vi "Main.vi"() -> ()   [LabVIEW 2019]
uses:
  Typedefs/#enum_State.ctl
  <vilib>/sound2/lvsound2.llb/Sound Data Format.ctl
  <vilib>/sound2/lvsound2.llb/Sampling Mode.ctl
  Typedefs/#cluster_ApplicationData.ctl
  <vilib>/sound2/lvsound2.llb/Sound File Refnum.ctl
  <vilib>/sound2/lvsound2.llb/Sound Input Task ID.ctl
  <vilib>/Utility/sysdir.llb/System Directory Type.ctl
  <vilib>/sound2/lvsound2.llb/Sound Input Read (DBL).vi
panel:
  in  "Record":bool
  out "Raw Data":waveform(dbl)[](graph)
  out "Spectrum Data":cluster{"f0":dbl, "df":dbl, "magnitude":dbl[]}[](graph)
  out "Threshold Exceeded?":bool
  in  "Threshold, dB":dbl=-100.0 format="%#_13g"
  in  "Upper Fc":dbl=3500.0 format="%#_13g"
  in  "Lower Fc":dbl=300.0 format="%#_13g"
  in  "Order":i32=6
  in  "Type":T1(ring)
  in  "Stop":bool
  # "FILTER SETTINGS"
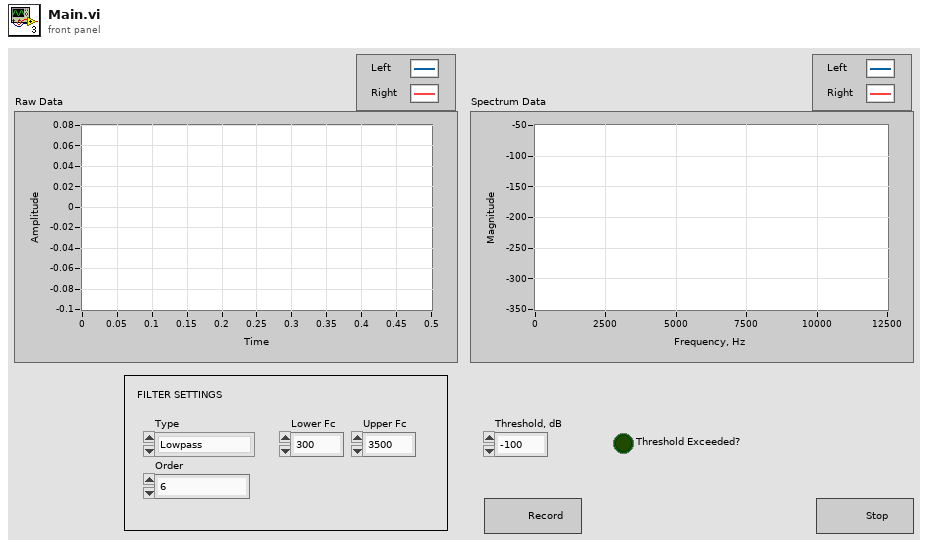
[diagram p1: front panel]
types:
  T1 = enum16{"Lowpass", "Highpass", "Bandpass", "Bandstop"}
  T2 = typedef "#enum_State.ctl" = enum16{"Init", "Acquisition", "Error Handler", "Exit", "Idle"}
  T3 = enum16{"open", "replace", "create", "open or create", "replace or create", "replace or create with confirmation"}
  T4 = typedef "Sound Data Format.ctl" = cluster{"sample rate (S/s)":dbl, "number of channels":i32, "bits per sample":i32}
  T5 = typedef "#cluster_ApplicationData.ctl" = cluster{"Sound file refnum":T6, "Acquisition task ID":T7, "Sound format":T4, "Number of samples/channel":i32, "Logging file refnum":refnum<file>}
  T6 = typedef "Sound File Refnum.ctl" = refnum<file>
  T7 = typedef "Sound Input Task ID.ctl" = u32
  T8 = typedef "System Directory Type.ctl" = i32
  T9 = typedef "Sampling Mode.ctl" = i32
  T10 = cluster{"Topology":enum16{"Off", "Butterworth", "Chebyshev", "Inverse Chebyshev", "Elliptic", "Bessel"}, "Type":enum16{"Lowpass", "Highpass", "Bandpass", "Bandstop"}, "Order":i32, "Lower Fc":dbl, "Upper Fc":dbl, "PB Ripple":dbl, "SB Attenuation":dbl}
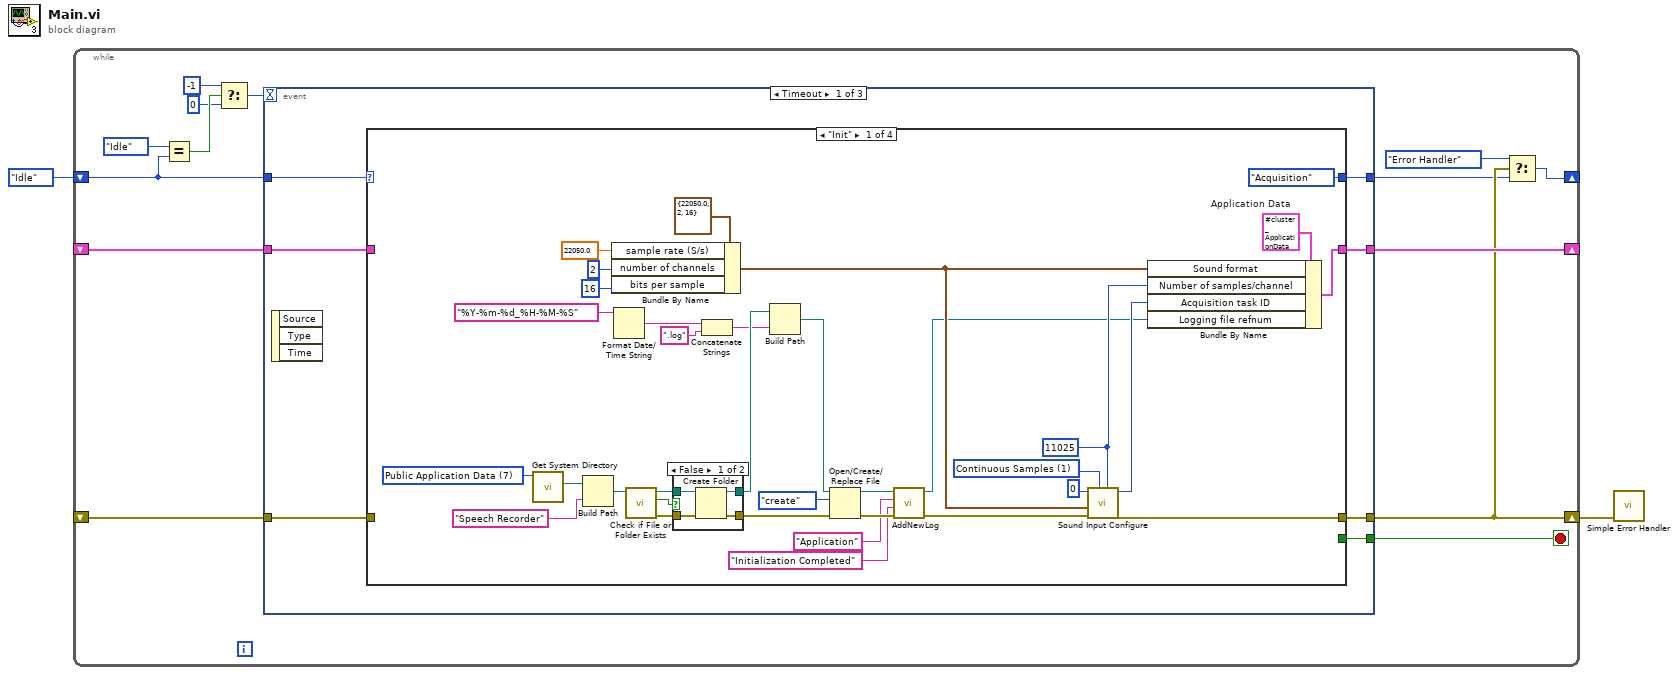
[diagram p0: block diagram]
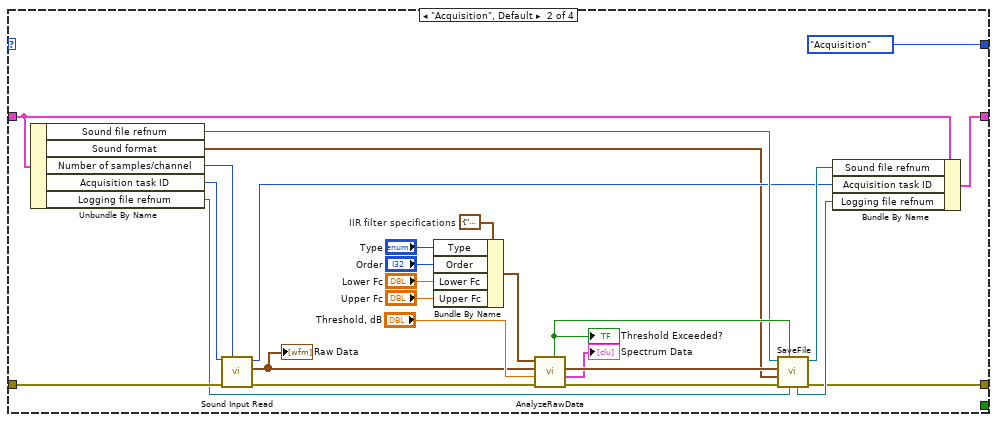
[diagram p3: hidden frame]
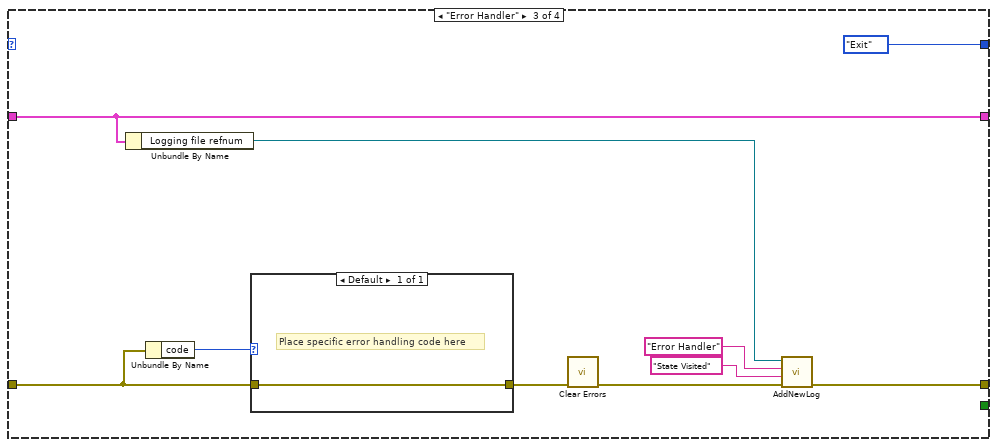
[diagram p4: hidden frame]
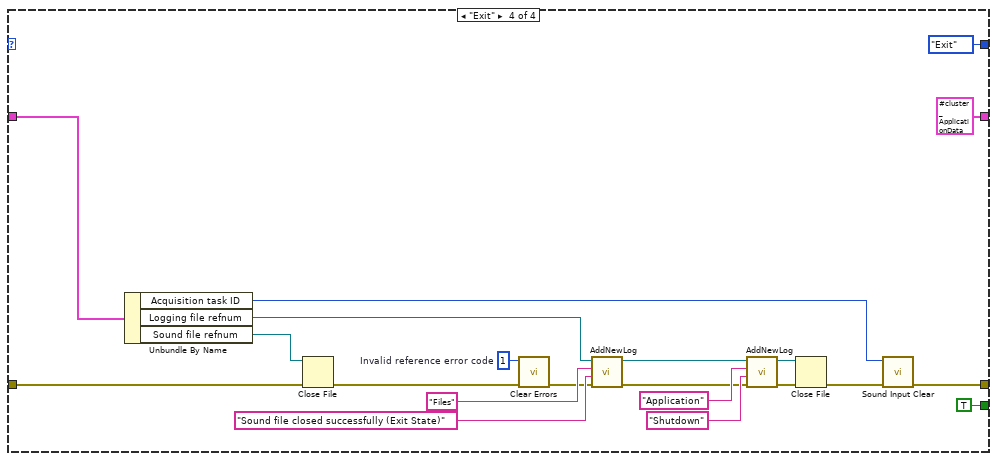
[diagram p5: hidden frame]
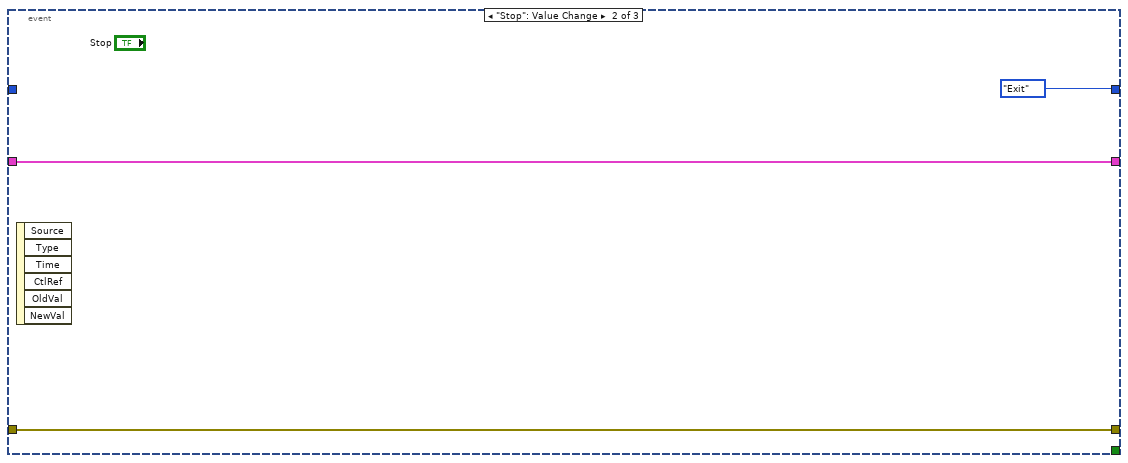
[diagram p6: hidden frame]
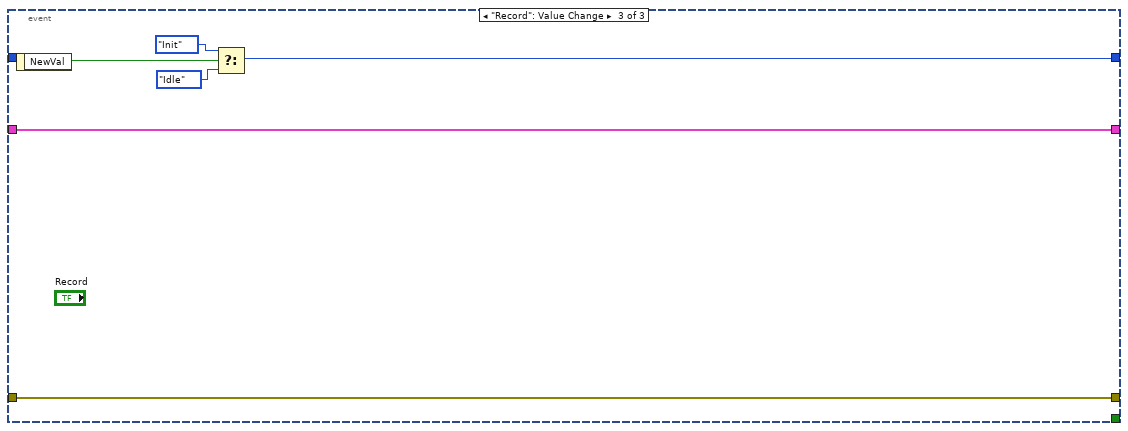
[diagram p7: hidden frame]
diagram:
  n1 = while {
    shift-right: [w9] -> _
    shift-left: #enum_State."Idle" ("State") -> [w8]
    shift-right: [w15] -> _
    shift-left: _ -> [w16]
    shift-right: [w12] -> w2
    shift-left: _ -> [w14]
    stop <- w13 stop-if-true
    n2 = Equal?(x=#enum_State."Idle", y=w8) -> (x = y?=w6:bool)
    n3 = Select(t=-1, s=w6, f=0) -> (s? t:f=w3:i32)
    n4 = event shown="[0] Timeout" {
      selector: _ -> [_ _ _]
      dyn-events: _ -> [_ _ _]
      timeout: w3 -> [_ _ _]
      tunnel: w8 -> [w23 _ _]
      tunnel: w16 -> [w22 w124 w130]
      tunnel: [w21 w124 w130] -> w15
      tunnel: w14 -> [w20 w123 w129]
      tunnel: [w19 _ _] -> w13
      tunnel: [w18 w123 w129] -> w12
      tunnel: [w17 #enum_State."Exit" ("State") w125] -> w10
      event Timeout {
        n5 = event-data() -> ()  [unwired: 1 in, 3 out]
        n6 = case shown="\"Init\"" w23 {
          tunnel: w20 -> [_ w89 w90 w121]
          tunnel: [w24 w64 w97 w104] -> w18
          tunnel: w22 -> [_ w74 w94 w118]
          tunnel: [w50 w73 w94 T5 {"Sound file refnum"=refnum, "Acquisition task ID"=0, "Sound format"={"sample rate (S/s)"=22050.0, "number of channels"=2, "bits per sample"=16}, "Number of samples/channel"=0, "Logging file refnum"=refnum} ("Application Data")] -> w21
          tunnel: [#enum_State."Acquisition" ("State") #enum_State."Acquisition" ("State") #enum_State."Exit" ("State") #enum_State."Exit" ("State")] -> w17
          tunnel: [_ _ _ TRUE] -> w19
          frame "Init" {
            w45 = T8 7 items=["User Home"=0, "User Desktop"=1, "User Documents"=2, "User Application Data"=3, "User Preferences"=4, "User Temporary"=5, "Public Documents"=6, "Public Application Data"=7, "Public Preferences"=8, "Public Cache"=13, "System Core Libraries"=9, "System Installed Libraries"=10, "Application Files"=11, "Boot Volume Root"=12] ("system directory type")
            w51 = T5 {"Sound file refnum"=refnum, "Acquisition task ID"=0, "Sound format"={"sample rate (S/s)"=22050.0, "number of channels"=2, "bits per sample"=16}, "Number of samples/channel"=0, "Logging file refnum"=refnum}  # Application Data
            w47 = 11025 ("Number of Samples/ch")
            w57 = T9 1 items=["Finite Samples", "Continuous Samples"] ("sample mode")
            n7 = call <vilib>:"Get System Directory.vi"("system directory type"=w45) -> ("system directory"=w44:path)  [unwired: 10 in]
            n8 = Build Path(base path=w44, name or relative path="Speech Recorder") -> (appended path=w42:path)
            n9 = Bundle By Name(cluster=T4 {"sample rate (S/s)"=22050.0, "number of channels"=2, "bits per sample"=16} ("sound format"), "sample rate (S/s)"=22050.0 ("Sample rate (Hz)"), "number of channels"=2 ("#Channels"), "bits per sample"=16 ("Resolution (bits)")) -> (w49:T4)
            n10 = Format Date/Time String(time format string (%c)="%Y-%m-%d_%H-%M-%S") -> (date/time string=w37:string)  [unwired: 2 in]
            n11 = call <vilib>:"Check if File or Folder Exists.vi"("path"=w42) -> ("error out"=w41:errorcluster, "file or folder exists?"=w39:bool, "dup path"=w40:path)  [unwired: 8 in]
            n12 = case shown="False" w39 {
              tunnel: w41 -> [w61 w62]
              tunnel: [w60 w62] -> w32
              tunnel: w40 -> [w59 w63]
              tunnel: [w58 w63] -> w38
              frame False {
                n13 = Create Folder(path (use dialog)=w59, error in=w61) -> (created path=w58:path, error out=w60:errorcluster)  [unwired: 1 in, 1 out]
              }
              frame True {
              }
            }
            n14 = Concatenate Strings(w37, ".log" ("string")) -> (w34:string)
            n15 = Build Path(base path=w38, name or relative path=w34) -> (appended path=w31:path)
            n16 = Open/Create/Replace File(file path (use dialog)=w31, error in=w32, operation (0:open)=T3."create") -> (refnum out=w28:refnum<file>, error out=w30:errorcluster)  [unwired: 3 in, 1 out]
            n17 = call "AddNewLog.vi"("error in"=w30, "Details"="Initialization Completed", "General Info"="Application", "Logging file refnum in"=w28) -> ("error out"=w29:errorcluster, "Logging file refnum out"=w27:refnum<file>)  [unwired: 6 in]
            n18 = call <vilib>:"Sound Input Configure.vi"("number of samples/ch"=w47, "sample mode"=w57, "error in (no error)"=w29, "sound format"=w49, "device ID"=u32 0 ("Device")) -> ("error out"=w24:errorcluster, "task ID"=w48:T7)  [unwired: 5 in]
            n19 = Bundle By Name(cluster=w51, "Sound format"=w49, "Number of samples/channel"=w47, "Acquisition task ID"=w48, "Logging file refnum"=w27) -> (w50:T5)
          }
          frame "Acquisition", Default {
            w88 = T10 {"Topology"=enum."Butterworth", "Type"=enum."Lowpass", "Order"=1, "Lower Fc"=100.0, "Upper Fc"=200.0, "PB Ripple"=1.0, "SB Attenuation"=60.0}  # IIR filter specifications
            n20 = Unbundle By Name(w74) -> ("Sound file refnum"=w75:T6, "Sound format"=w68:T4, "Number of samples/channel"=w69:i32, "Acquisition task ID"=w70:T7, "Logging file refnum"=w65:refnum<file>)
            n21 = call-poly <vilib>:"Sound Input Read.vi"("number of samples/ch"=w69, "error in (no error)"=w89, "task ID"=w70) -> ("error out"=w83:errorcluster, "data"=w81:waveform(dbl)[], "task ID out"=w71:T7)  [unwired: 6 in]
            "Raw Data" <- w81
            n22 = Bundle By Name(cluster=w88, "Type"="Type", "Order"="Order", "Lower Fc"="Lower Fc", "Upper Fc"="Upper Fc") -> (w80:T10)
            n23 = call "AnalyzeRawData.vi"("error in (no error)"=w83, "Threshold, dB"="Threshold, dB", "Raw Data"=w81, "IIR Filter Specifications"=w80) -> ("error out"=w77:errorcluster, "Power Spectrum / PSD"=→"Spectrum Data":cluster{"f0":dbl, "df":dbl, "magnitude":dbl[]}[], "Filtered Data"=w79:waveform(dbl)[], "Threshold Exceeded?"=w76:bool)  [unwired: 4 in]
            "Threshold Exceeded?" <- w76
            n24 = call "SaveFile.vi"("Logging file refnum in"=w65, "Threshold Exceeded?"=w76, "Error in"=w77, "Sound format"=w68, "Filtered Data"=w79, "Sound file refnum in"=w75) -> ("Error out"=w64:errorcluster, "Sound file refnum out"=w72:T6, "Logging file refnum out"=w66:refnum<file>)  [unwired: 3 in]
            n25 = Bundle By Name(cluster=w74, "Sound file refnum"=w72, "Acquisition task ID"=w71, "Logging file refnum"=w66) -> (w73:T5)
          }
          frame "Error Handler" {
            n26 = Unbundle By Name(w94) -> ("Logging file refnum"=w93:refnum<file>)
            n27 = Unbundle By Name(w90) -> ("code"=w92:i32)
            n28 = case shown="Default" w92 {
              tunnel: [w100] -> w91
              tunnel: w90 -> [w100]
              frame Default {
                # "Place specific error handling code here"
              }
            }
            n29 = call <vilib>:"Clear Errors.vi"("error in (no error)"=w91) -> ("error out"=w99:errorcluster)  [unwired: 5 in, 1 out]
            n30 = call "AddNewLog.vi"("error in"=w99, "Details"="State Visited" ("string"), "General Info"="Error Handler" ("string"), "Logging file refnum in"=w93) -> ("error out"=w97:errorcluster)  [unwired: 6 in, 1 out]
          }
          frame "Exit" {
            w101 = 1  # Invalid reference error code
            n31 = Unbundle By Name(w118) -> ("Acquisition task ID"=w106:T7, "Logging file refnum"=w110:refnum<file>, "Sound file refnum"=w111:T6)
            n32 = Close File(refnum=w111, error in=w121) -> (error out=w103:errorcluster)  [unwired: 1 out]
            n33 = call <vilib>:"Clear Errors.vi"("error in (no error)"=w103, "specific error code to clear (0: all)"=w101) -> ("error out"=w102:errorcluster)  [unwired: 4 in, 1 out]
            n34 = call "AddNewLog.vi"("error in"=w102, "Details"="Sound file closed successfully (Exit State)" ("string"), "General Info"="Files" ("string"), "Logging file refnum in"=w110) -> ("error out"=w112:errorcluster, "Logging file refnum out"=w109:refnum<file>)  [unwired: 6 in]
            n35 = call "AddNewLog.vi"("error in"=w112, "Details"="Shutdown" ("General Info"), "General Info"="Application", "Logging file refnum in"=w109) -> ("error out"=w116:errorcluster, "Logging file refnum out"=w115:refnum<file>)  [unwired: 6 in]
            n36 = Close File(refnum=w115, error in=w116) -> (error out=w105:errorcluster)  [unwired: 1 out]
            n37 = call <vilib>:"Sound Input Clear.vi"("error in (no error)"=w105, "task ID"=w106) -> ("error out"=w104:errorcluster)  [unwired: 9 in]
          }
        }
      }
      event "Stop": Value Change {
        n38 = event-data() -> ()  [unwired: 1 in, 6 out]
      }
      event "Record": Value Change {
        n39 = event-data() -> ("NewVal"=w128:bool)  [unwired: 1 in]
        n40 = Select(t=#enum_State."Init" ("State"), s=w128, f=#enum_State."Idle" ("State")) -> (s? t:f=w125:T2)
      }
    }
    n41 = Select(t=#enum_State."Error Handler" ("State"), s=w12, f=w10) -> (s? t:f=w9:T2)
  }
  n42 = call <vilib>:"Simple Error Handler.vi"("error in (no error)"=w2) -> ()  [unwired: 4 in, 5 out]
